vi "Highlight Object.vi"(8 "Error In":errorcluster, 10 "Tag":string, 11 "Bookmarks":T1[](array[typedef])) -> (0 "Error Out":errorcluster)   [LabVIEW 2017, in "Bookmark Manager.lvlib"]
uses:
  Bookmark Manager.lvlib
  VI Bookmark.ctl
  VI Information.ctl
  Application Information.ctl
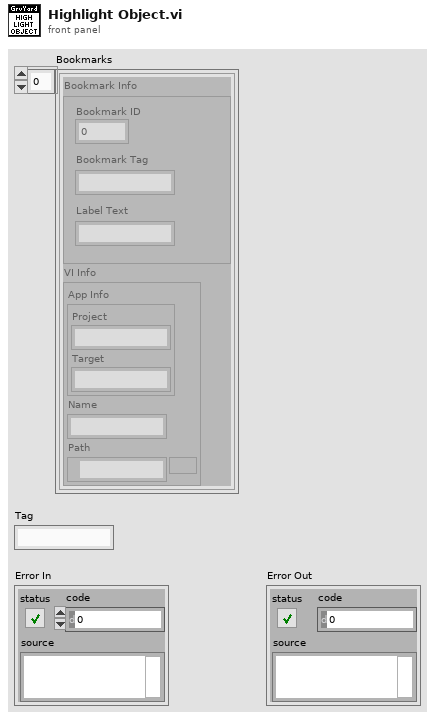
[diagram p1: front panel]
types:
  T1 = typedef "Bookmark Manager.lvlib/VI Bookmark.ctl" = cluster{"Bookmark Info":cluster{"Bookmark ID":u32, "Bookmark Tag":string, "Label Text":string}, "VI Info":T2}
  T2 = typedef "Bookmark Manager.lvlib/VI Information.ctl" = cluster{"App Info":T3, "Name":string, "Path":path}
  T3 = typedef "Bookmark Manager.lvlib/Application Information.ctl" = cluster{"Project":string, "Target":string}
  T4 = enum32{"Bad", "Idle", "Run top level", "Running"}
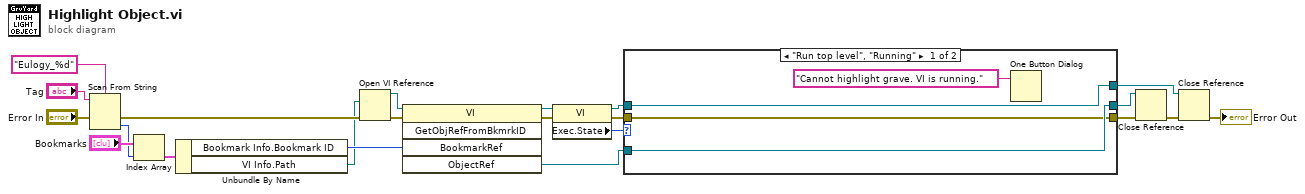
[diagram p0: block diagram]
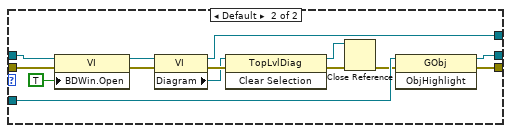
[diagram p2: hidden frame]
diagram:
  n1 = Scan From String(format string="Eulogy_%d", input string="Tag", error in="Error In") -> (error out=w21:errorcluster, output 1=w17:i32)  [unwired: 2 in, 2 out]
  n2 = Index Array(array="Bookmarks", index=w17) -> (element=w3:T1)
  n3 = Unbundle By Name(w3) -> ("Bookmark Info.Bookmark ID"=w2:u32, "VI Info.Path"=w1:path)
  n4 = Open VI Reference(vi path=w1, error in (no error)=w21) -> (vi reference=w15:refnum<vi>, error out=w16:errorcluster)  [unwired: 4 in]
  n5 = invoke class="VI" method="GetObjRefFromBkmrkID"(reference=w15, error in=w16, "BookmarkRef"=w2) -> (reference out=w13:refnum<vi>, error out=w14:errorcluster, "ObjectRef"=w9:refnum<vi>)  [unwired: 2 in, 2 out]
  n6 = property class="VI"(reference=w13, error in=w14) -> (reference out=w8:refnum<vi>, error out=w11:errorcluster, "Exec.State"=w12:T4)
  n7 = case shown="\"Run top level\", \"Running\"" w12 {
    tunnel: [w24 w37] -> w10
    tunnel: w11 -> [w24 w33]
    tunnel: w9 -> [w25 w40]
    tunnel: w8 -> [w26 w38]
    tunnel: [w26 w27] -> w6
    tunnel: [w25 w39] -> w4
    frame "Run top level", "Running" {
      n8 = One Button Dialog(message="Cannot highlight grave. VI is running.") -> ()  [unwired: 1 in, 1 out]
    }
    frame Default {
      n9 = property class="VI"(reference=w38, error in=w33, "BDWin.Open"=TRUE ("Block Diagram Window:Open")) -> (reference out=w34:refnum<vi>, error out=w32:errorcluster)
      n10 = property class="VI"(reference=w34, error in=w32) -> (reference out=w27:refnum<vi>, error out=w36:errorcluster, "Diagram"=w35:refnum<vi>)
      n11 = invoke class="TopLvlDiag" method="Clear Selection"(reference=w35, error in=w36) -> (reference out=w30:refnum<vi>, error out=w29:errorcluster)  [unwired: 1 in, 1 out]
      n12 = Close Reference(reference=w30, error in (no error)=w29) -> (error out=w28:errorcluster)
      n13 = invoke class="GObj" method="ObjHighlight"(reference=w40, error in=w28) -> (reference out=w39:refnum<vi>, error out=w37:errorcluster)  [unwired: 1 in, 1 out]
    }
  }
  n14 = Close Reference(reference=w4, error in (no error)=w10) -> (error out=w5:errorcluster)
  n15 = Close Reference(reference=w6, error in (no error)=w5) -> (error out=→"Error Out":errorcluster)
